vi "When Method One Return Value.vi"(0 "error out":errorcluster, 2 "Return Value":dbl, 8 "error in (no error)":errorcluster, 11 "Test Interface Mock In":refnum<class "Test Interface Responsive Mock.lvclass">) -> (3 "Test Interface Mock Out":refnum<class "Test Interface Responsive Mock.lvclass">)   [LabVIEW 2020, in "Test Interface Responsive Mock.lvclass"]
uses:
  Test Interface Responsive Mock.lvclass
  C:/git/astemes-lmock/source/Framework/Responsive Mock/Responsive Mock.lvclass
  source/Framework/Responsive Mock/Responsive Mock.lvclass
panel:
  # "Important"
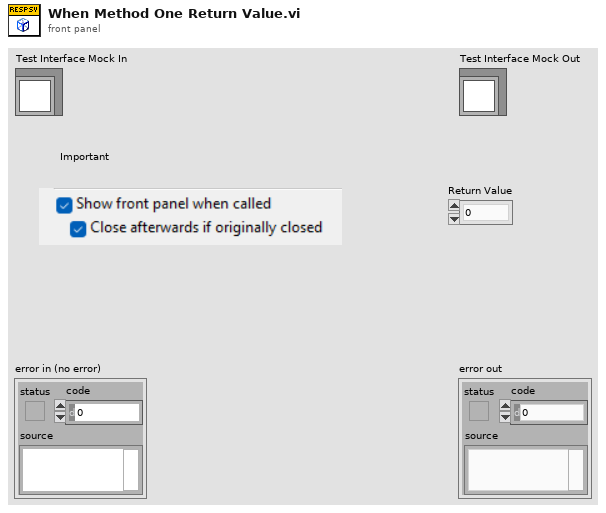
[diagram p1: front panel]
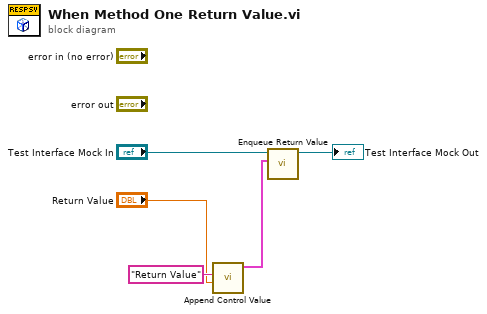
[diagram p0: block diagram]
diagram:
  n1 = call "Append Control Value.vi"("Variant Data"="Return Value", "Name"="Return Value") -> ("Control Values"=w1:cluster{"Name":string, "Variant Data":variant}[])  [unwired: 9 in]
  n2 = call "Enqueue Return Value.vi"("Indicator Values"=w1, "Mock In"="Test Interface Mock In") -> ("Mock Out"=→"Test Interface Mock Out":refnum<class "Test Interface Responsive Mock.lvclass">)  [unwired: 8 in, 1 out]
